vi "Periodic Tasks.vi"(8 "error in":errorcluster) -> ()   [LabVIEW 2019]
doc: "This VI runs in parallel to other tasks. It can contain as many user-defined periodic loops as you need. These can carry out PID or other sorts of timed response."
uses:
  <vilib>/Rock Robotics/WPI/Utilities/WPI_GetSetVariantRefNum.vi
  Robot Global Data.vi
  <vilib>/Rock Robotics/WPI/RobotDrive/WPI_RobotDriveArcadeDrive_Standard(NoSaturation).vi
  <vilib>/Rock Robotics/Network Tables/NT Read Number.vi
  <vilib>/Rock Robotics/Network Tables/NT Write Numeric Array.vi
  <vilib>/Rock Robotics/Network Tables/NT Read Boolean.vi
panel:
  in  "Proportional Gain":dbl=0.25
  in  "Target X":dbl=0.5
  out "output":T1
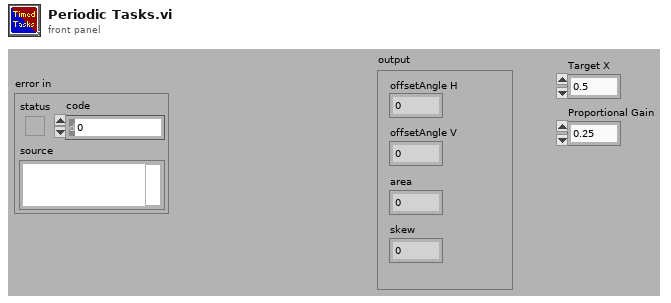
[diagram p1: front panel]
types:
  T1 = cluster{"offsetAngle H":dbl, "offsetAngle V":dbl, "area":dbl, "skew":dbl}
  T2 = typedef "WPI_JoystickDevRef.ctl" = cluster{"Device":T3}
  T3 = typedef "WPI_JoystickDeviceEnum.ctl" = enum16{"USB 0", "USB 1", "USB 2", "USB 3", "USB 4", "USB 5"}
  T4 = typedef "WPI_RobotDriveDevRef.ctl" = cluster{"DevStatus":errorcluster, "Motors[]":T5[], "Square Inputs":bool, "Max Output":dbl}
  T5 = typedef "WPI_MotorControlDeviceRef.ctl" = cluster{"DeviceStatus":errorcluster, "Type":T6, "PWM":cluster{"PWM Channel":T7, "DeadBand":T8}, "CAN":cluster{"Device Number":u8, "SetOutput VI Ref":variant, "GetOutput VI Ref":variant, "Enable VI Ref":variant, "Disable VI Ref":variant, "Data":variant}, "Invert":bool, "DIO PWM":cluster{"PWM \"Enable\" Channel":T7, "DIOChannel":T9, "PWM Rate":dbl}}
  T6 = typedef "WPI_MotorControlType.ctl" = enum16{"PWM", "CAN", "DIO PWM"}
  T7 = typedef "FPGA_DIOPWMChannel.ctl" = enum8{"PWM 0", "PWM 1", "PWM 2", "PWM 3", "PWM 4", "PWM 5", "PWM 6", "PWM 7", "PWM 8", "PWM 9", "PWM MXP 0", "PWM MXP 1", "PWM MXP 2", "PWM MXP 3", "PWM MXP 4", "PWM MXP 5", "PWM MXP 6", "PWM MXP 7", "PWM MXP 8", "PWM MXP 9", "Invalid"}
  T8 = typedef "WPI_PWMDeadband.ctl" = cluster{"Name":string, "maxPositivePwm":i32, "minPositivePwm":i32, "centerPwm":i32, "maxNegativePwm":i32, "minNegativePwm":i32, "angularRange":u16}
  T9 = typedef "FPGA_DIOChannel.ctl" = enum8{"DIO 0", "DIO 1", "DIO 2", "DIO 3", "DIO 4", "DIO 5", "DIO 6", "DIO 7", "DIO 8", "DIO 9", "DIO MXP 0", "DIO MXP 1", "DIO MXP 2", "DIO MXP 3", "DIO MXP 4", "DIO MXP 5", "DIO MXP 6", "DIO MXP 7", "DIO MXP 8", "DIO MXP 9", "DIO MXP 10", "DIO MXP 11", "DIO MXP 12", "DIO MXP 13", "DIO MXP 14", "DIO MXP 15", "SPI Port CS1", "SPI Port CS2", "SPI Port CS3", "SPI Port MISO", "SPI Port MOSI", "Invalid"}
  T10 = cluster{"JoystickDevRef":T2, "RobotDriveDevRef":T4}
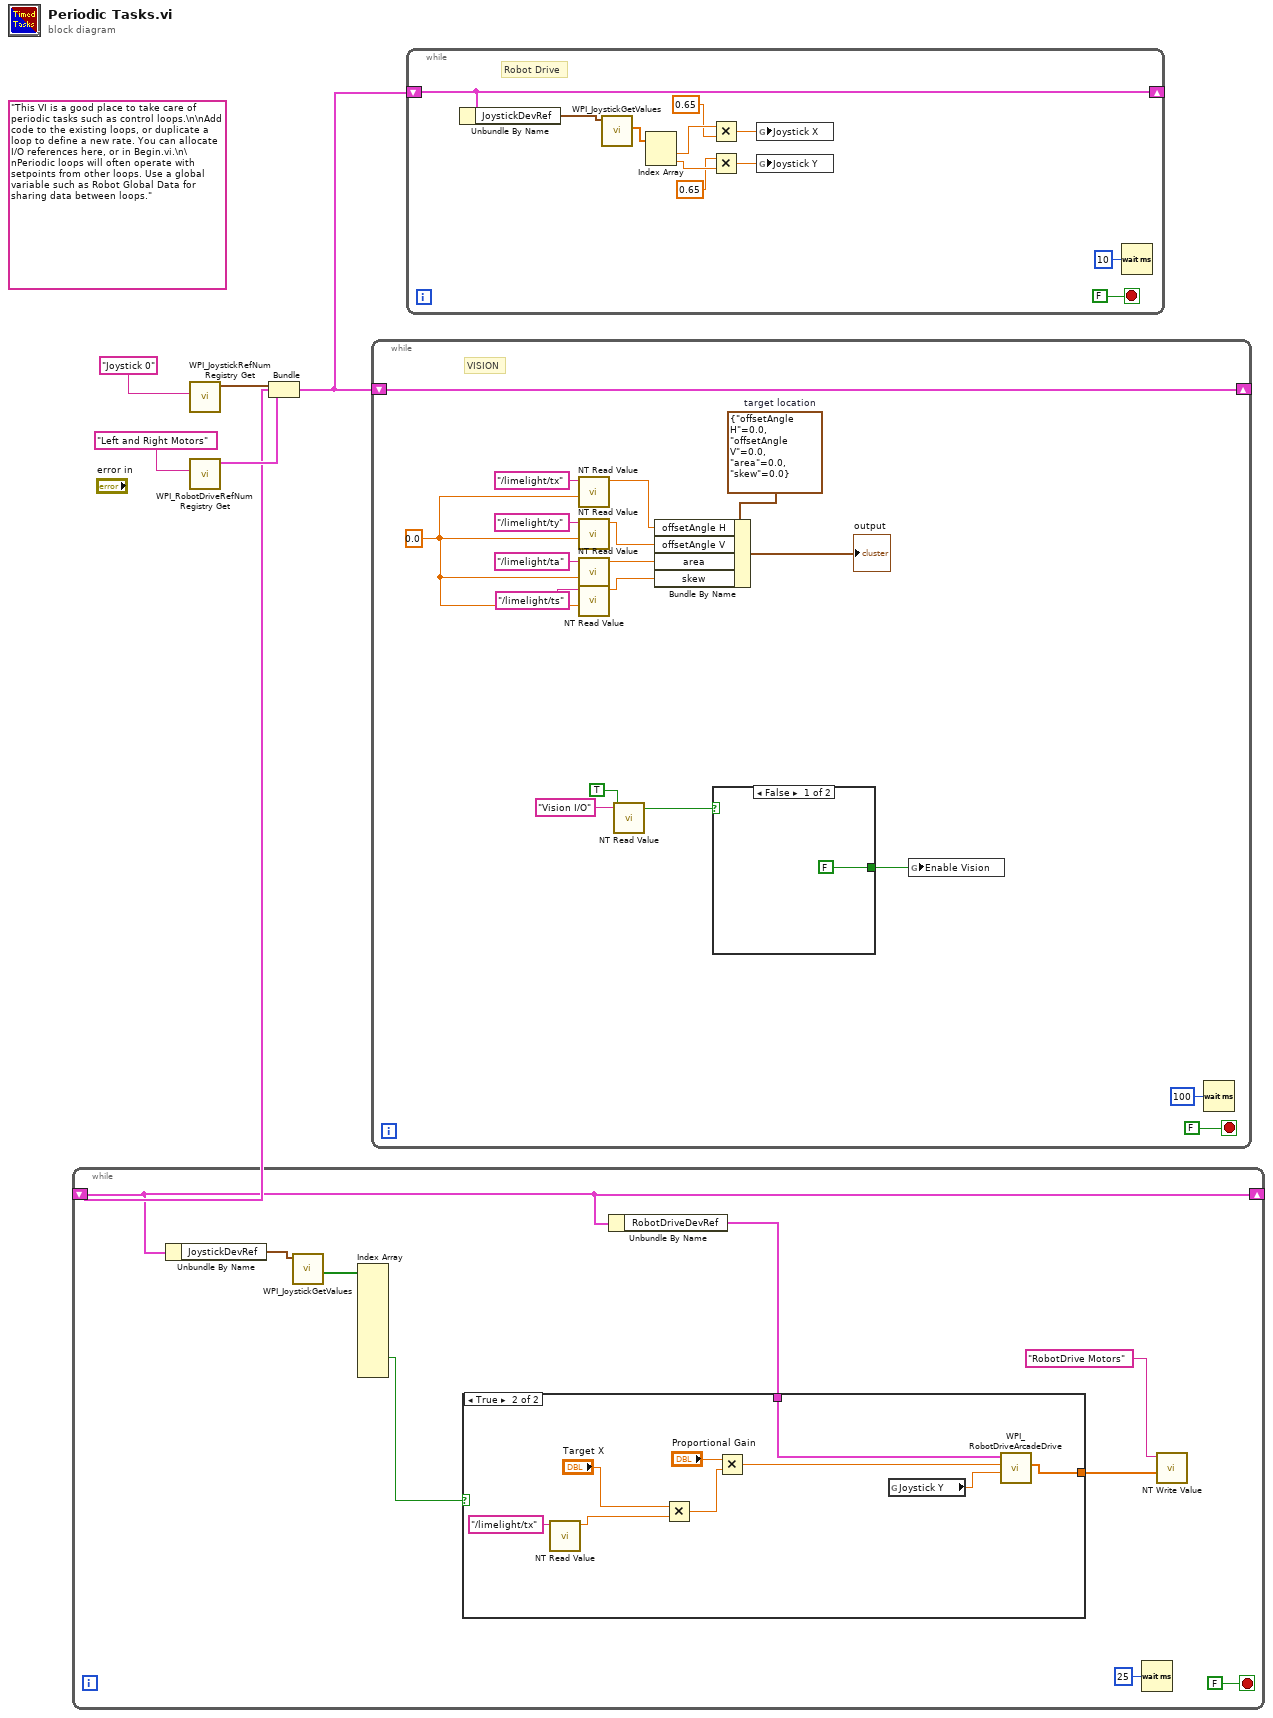
[diagram p0: block diagram]
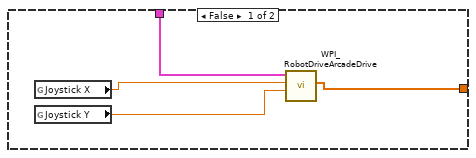
[diagram p2: hidden frame]
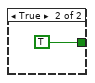
[diagram p3: hidden frame]
diagram:
  (unwired) "This VI is a good place to take care of periodic tasks such as control loops.\n\nAdd code to the existing loops, or duplicate a loop to define a new rate. You can allocate I/O references here, or in Begin.vi.\n\nPeriodic loops will often operate with setpoints from other loops. Use a global variable such as Robot Global Data for sharing data between loops."
  n1 = call <vilib>:"WPI_JoystickRefNum Registry Get.vi"("refnum name"="Joystick 0") -> ("JoystickDevRef"=w3:T2)  [unwired: 1 in, 9 out]
  n2 = call <vilib>:"WPI_RobotDriveRefNum Registry Get.vi"("refnum name"="Left and Right Motors") -> ("RobotDriveDevRef"=w2:T4)  [unwired: 1 in, 9 out]
  n3 = Bundle("JoystickDevRef"=w3, "RobotDriveDevRef"=w2) -> (w1:T10)  [unwired: 1 out]
  n4 = while {
    shift-right: [w12] -> _
    shift-left: w1 -> [w12]
    stop <- FALSE stop-if-true
    n5 = Unbundle By Name(w12) -> ("JoystickDevRef"=w11:T2)
    n6 = call <vilib>:"WPI_JoystickGetValues.vi"("JoystickDevRef"=w11) -> ("Buttons"=w10:bool[])  [unwired: 6 in, 4 out]
    n7 = Index Array(array=w10) -> (element #10=w6:bool)  [unwired: 12 in, 11 out]
    n8 = Unbundle By Name(w12) -> ("RobotDriveDevRef"=w9:T4)
    n9 = case shown="True" w6 {
      tunnel: w9 -> [w18 w27]
      tunnel: [w15 w19] -> w7
      frame False {
        n10 = global read "Robot Global Data.vi" "Joystick X"() -> (w17:dbl)
        n11 = global read "Robot Global Data.vi" "Joystick Y"() -> (w16:dbl)
        n12 = call-poly <vilib>:"WPI_RobotDriveArcadeDrive.vi"("Y axis value"=w16, "X axis value"=w17, "RobotDriveDevRef"=w18) -> ("Motor Values"=w15:dbl[])  [unwired: 6 in, 2 out]
      }
      frame True {
        n13 = call-poly <vilib>:"NT Read Value.vi"("Name"="/limelight/tx") -> ("Numeric"=w25:dbl)  [unwired: 9 in, 1 out]
        n14 = Multiply(x="Target X", y=w25) -> (x*y=w23:dbl)
        n15 = Multiply(x="Proportional Gain", y=w23) -> (x*y=w21:dbl)
        n16 = global read "Robot Global Data.vi" "Joystick Y"() -> (w20:dbl)
        n17 = call-poly <vilib>:"WPI_RobotDriveArcadeDrive.vi"("Y axis value"=w20, "X axis value"=w21, "RobotDriveDevRef"=w27) -> ("Motor Values"=w19:dbl[])  [unwired: 6 in, 2 out]
      }
    }
    n18 = Wait (ms)(milliseconds to wait=u32 25) -> ()  [unwired: 1 out]
    n19 = call-poly <vilib>:"NT Write Value.vi"("Numeric Array"=w7, "Name"="RobotDrive Motors") -> ()  [unwired: 9 in, 1 out]
  }
  n20 = while {
    shift-right: [w32] -> _
    shift-left: w1 -> [w32]
    stop <- FALSE stop-if-true
    w33 = 0.0
    w42 = T1 {"offsetAngle H"=0.0, "offsetAngle V"=0.0, "area"=0.0, "skew"=0.0}  # target location
    # "VISION"
    n21 = call-poly <vilib>:"NT Read Value.vi"("Default Value"=w33, "Name"="/limelight/tx") -> ("Numeric"=w38:dbl)  [unwired: 8 in, 1 out]
    n22 = call-poly <vilib>:"NT Read Value.vi"("Default Value"=w33, "Name"="/limelight/ty") -> ("Numeric"=w39:dbl)  [unwired: 8 in, 1 out]
    n23 = call-poly <vilib>:"NT Read Value.vi"("Default Value"=w33, "Name"="/limelight/ta") -> ("Numeric"=w40:dbl)  [unwired: 8 in, 1 out]
    n24 = call-poly <vilib>:"NT Read Value.vi"("Default Value"=w33, "Name"="/limelight/ts") -> ("Numeric"=w41:dbl)  [unwired: 8 in, 1 out]
    n25 = call-poly <vilib>:"NT Read Value.vi"("Default Value"=TRUE, "Name"="Vision I/O") -> ("Boolean"=w29:bool)  [unwired: 8 in, 1 out]
    n26 = Bundle By Name(cluster=w42, "offsetAngle H"=w38, "offsetAngle V"=w39, "area"=w40, "skew"=w41) -> (→"output":T1)
    n27 = case shown="False" w29 {
      tunnel: [FALSE ("Enable Vision") TRUE ("Enable Vision")] -> w28
      frame False {
      }
      frame True {
      }
    }
    n28 = global write "Robot Global Data.vi" "Enable Vision"(w28) -> ()
    n29 = Wait (ms)(milliseconds to wait=u32 100) -> ()  [unwired: 1 out]
  }
  n30 = while {
    shift-right: [w56] -> _
    shift-left: w1 -> [w56]
    stop <- FALSE stop-if-true
    # "Robot Drive"
    n31 = Unbundle By Name(w56) -> ("JoystickDevRef"=w55:T2)
    n32 = call <vilib>:"WPI_JoystickGetValues.vi"("JoystickDevRef"=w55) -> ("Axes"=w54:dbl[])  [unwired: 6 in, 4 out]
    n33 = Index Array(array=w54) -> (element #1=w53:dbl, element #2=w51:dbl)  [unwired: 2 in]
    n34 = Multiply(x=w53, y=0.65) -> (x*y=w49:dbl)
    n35 = Multiply(x=0.65, y=w51) -> (x*y=w48:dbl)
    n36 = global write "Robot Global Data.vi" "Joystick X"(w49) -> ()
    n37 = global write "Robot Global Data.vi" "Joystick Y"(w48) -> ()
    n38 = Wait (ms)(milliseconds to wait=u32 10) -> ()  [unwired: 1 out]
  }
